vi "WinkelGeschwindigkeit.vi"() -> ()   [LabVIEW 2013]
uses:
  <vilib>/DAQmx/read.llb/DAQmx Read (Counter DBL 1Chan 1Samp).vi
  <vilib>/DAQmx/configure/timing.llb/DAQmx Timing (Sample Clock).vi
  <vilib>/Platform/TimedLoop/XDataNode/XDataNode.xnode
  <vilib>/Platform/TimedLoop/XDataNode/nitl_modes.ctl
  <vilib>/Platform/TimedLoop/XDataNode/XDNodeRunTimeDep.lvlib
  <vilib>/Platform/TimedLoop/XDataNode/wakeup.ctl
  <vilib>/Platform/TimedLoop/XDataNode/timing_clust.ctl
panel:
  out "Signalverlaufsdiagramm":dbl(graph)
  out "error out":errorcluster caption="Fehler (Ausgang)"
  out "frequency":dbl caption="Frequenz"
  in  "Stopp":bool
  in  "error in":errorcluster caption="Fehler (Eingang)"
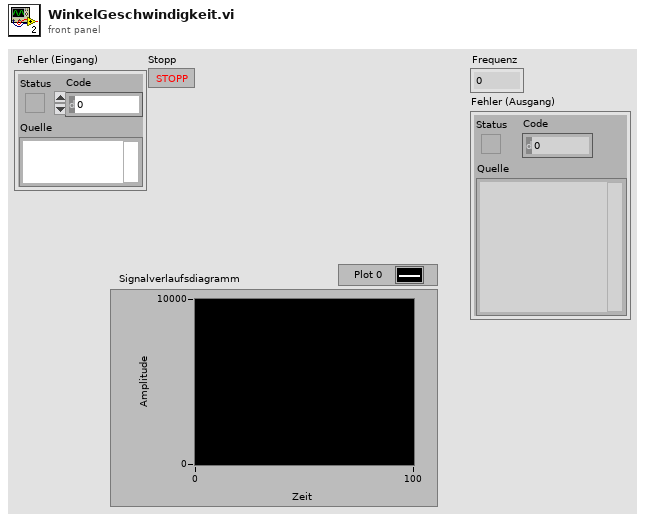
[diagram p1: front panel]
types:
  T1 = typedef "XDNodeRunTimeDep.lvlib/timing_clust.ctl" = cluster{"Expected End [f-1]":u64, "Actual End [f-1]":u64, "Finished Late? [f-1]":bool, "Expected End [i-1]":u64, "Actual End [i-1]":u64, "Finished Late? [i-1]":bool, "Expected Start [i]":u64, "Actual Start [i]":u64, "Expected Start [f]":u64, "Actual Start [f]":u64, "Source Name":string, "Structure Name":string, "Period":i64, "Deadline":i64, "Offset":i64, "Start":i64, "Priority":i32, "Timeout":i32, "Mode":T2, "Wakeup Reason":T3, "Error":errorcluster, "Source Type":string, "Secondary Source Type":string, "Global End Time":u64, "Global Start Time":u64, "Frame Duration":u64, "Iteration Duration":u64, "Assigned CPU":i32, "I/O Scan Engine Mode":u32}
  T2 = typedef "XDNodeRunTimeDep.lvlib/nitl_modes.ctl" = enum32{"No Change", "Process missed periods, maintain original phase", "Discard missed periods, maintain original phase", "Process missed periods, ignore original phase", "Discard missed periods, ignore original phase"}
  T3 = typedef "XDNodeRunTimeDep.lvlib/wakeup.ctl" = enum32{"Normal", "Aborted", "Asynchronous wakeup", "Timing source error", "Timed loop error", "Timeout"}
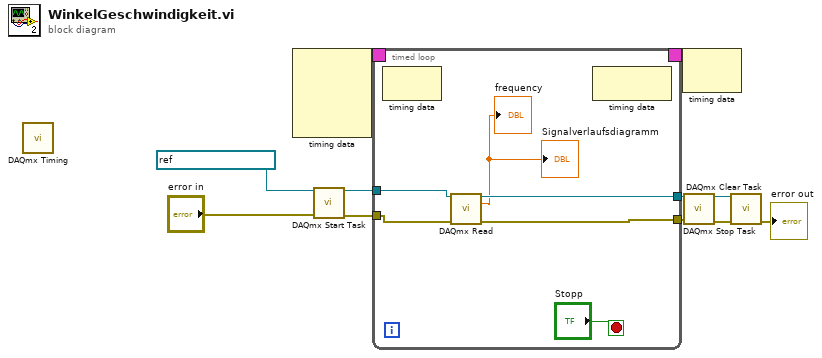
[diagram p0: block diagram]
diagram:
  n1 = call-poly <vilib>:"DAQmx Timing.vi"() -> ()  [unwired: 14 in, 2 out]
  n2 = node-c288() -> (w2:T1)  [unwired: 4 in]
  n3 = call <vilib>:"DAQmx Start Task.vi"("task/channels in"=refnum<k21> "EncoderFrequenz", "error in"="error in") -> ("task out"=w10:refnum<k21>, "error out"=w11:errorcluster)  [unwired: 12 in]
  n4 = timed-loop {
    tunnel: w11 -> [w16]
    tunnel: w10 -> [w15]
    tunnel: [w14] -> w6
    tunnel: [w13] -> w7
    timing: w2 -> [_]
    timing-out: [_] -> w1
    stop <- "Stopp" stop-if-true
    n5 = node-c288() -> ()  [unwired: 1 in, 1 out]
    n6 = call-poly <vilib>:"DAQmx Read.vi"("task/channels in"=w15, "error in"=w16) -> ("task out"=w14:refnum<k21>, "data"=→"frequency" →"Signalverlaufsdiagramm":dbl, "error out"=w13:errorcluster)  [unwired: 11 in]
    n7 = node-c288() -> ()  [unwired: 1 in, 1 out]
  }
  n8 = node-c288(w1) -> ()  [unwired: 1 out]
  n9 = call <vilib>:"DAQmx Stop Task.vi"("task/channels in"=w6, "error in"=w7) -> ("task out"=w9:refnum<k21>, "error out"=w8:errorcluster)  [unwired: 12 in]
  n10 = call <vilib>:"DAQmx Clear Task.vi"("task in"=w9, "error in"=w8) -> ("error out"=→"error out":errorcluster)  [unwired: 13 in]
